vi "全局配置.vi"() -> ()   [LabVIEW 2018]
uses:
  Settings/Settings.ctl
  Acquisition/Hardware Configuration.ctl
  Acquisition/Signal Type.ctl
  Acquisition/Acquisition.lvlib
  Settings/Settings.lvlib
panel:
  in  "配置":T1 {"串口通信UI"."Format" items=["标准帧", "扩展帧"]; "串口通信UI"."Type" items=["数据帧", "远程帧"]; "串口通信UI"."ID" format="0x%x"; "串口通信UI"."Fliter" items=["接收所有类型"=1, "只接收标准帧"=2, "只接收扩展帧"=3]; "串口通信UI"."kBaudRate" items=["5k bps"=1, "10k bps"=2, "20k bps"=3, "40k bps"=4, "50k bps"=5, "80k bps"=6, "100k bps"=7, "125k bps"=8, "200k bps"=9, "250k bps"=10, "400k bps"=11, "500k bps"=12, "666k bps"=13, "800k bps"=14, "1000k bps"=15, "33.33k bps"=16, "66.66k bps"=17, "83.33k bps"=18]; "串口通信UI"."Mode" items=["正常工作", "仅侦听模式", "自测模式（环回）"]; "串口通信UI"."InitFlag" items=["使用界面设置参数"=1]; "串口通信UI"."AccMask" format="%08x"; "串口通信UI"."AccCode" format="%08x"; "串口通信UI"."Channel" items=["通道1", "通道2"]; "串口通信UI"."DevType" items=["USB-CAN"=3, "USB-CAN2"=4]; "安全报警UI"."操作 8" items=["产生报警信息（不发声），等待手动操作", "产生报警信息（发声），等待手动操作", "产生报警信息（不发声），自动刹车", "产生报警信息（发声），自动刹车", "产生报警信息（不发声），立即自动断电，开启泄放电阻", "产生报警信息（发声），立即自动断电，开启泄放电阻"]; "安全报警UI"."操作 7" items=["产生报警信息（不发声），等待手动操作", "产生报警信息（发声），等待手动操作", "产生报警信息（不发声），自动刹车", "产生报警信息（发声），自动刹车", "产生报警信息（不发声），立即自动断电，开启泄放电阻", "产生报警信息（发声），立即自动断电，开启泄放电阻"]; "安全报警UI"."操作 6" items=["产生报警信息（不发声），等待手动操作", "产生报警信息（发声），等待手动操作", "产生报警信息（不发声），自动刹车", "产生报警信息（发声），自动刹车", "产生报警信息（不发声），立即自动断电，开启泄放电阻", "产生报警信息（发声），立即自动断电，开启泄放电阻"]; "安全报警UI"."操作 5" items=["产生报警信息（不发声），等待手动操作", "产生报警信息（发声），等待手动操作", "产生报警信息（不发声），自动刹车", "产生报警信息（发声），自动刹车", "产生报警信息（不发声），立即自动断电，开启泄放电阻", "产生报警信息（发声），立即自动断电，开启泄放电阻"]; "安全报警UI"."操作 4" items=["产生报警信息（不发声），等待手动操作", "产生报警信息（发声），等待手动操作", "产生报警信息（不发声），自动刹车", "产生报警信息（发声），自动刹车", "产生报警信息（不发声），立即自动断电，开启泄放电阻", "产生报警信息（发声），立即自动断电，开启泄放电阻"]; "安全报警UI"."操作 3" items=["产生报警信息（不发声），等待手动操作", "产生报警信息（发声），等待手动操作", "产生报警信息（不发声），自动刹车", "产生报警信息（发声），自动刹车", "产生报警信息（不发声），立即自动断电，开启泄放电阻", "产生报警信息（发声），立即自动断电，开启泄放电阻"]; "安全报警UI"."操作 2" items=["产生报警信息（不发声），等待手动操作", "产生报警信息（发声），等待手动操作", "产生报警信息（不发声），自动刹车", "产生报警信息（发声），自动刹车", "产生报警信息（不发声），立即自动断电，开启泄放电阻", "产生报警信息（发声），立即自动断电，开启泄放电阻"]; "安全报警UI"."操作" items=["产生报警信息（不发声），等待手动操作", "产生报警信息（发声），等待手动操作", "产生报警信息（不发声），自动刹车", "产生报警信息（发声），自动刹车", "产生报警信息（不发声），立即自动断电，开启泄放电阻", "产生报警信息（发声），立即自动断电，开启泄放电阻"]}
  # "参数配置文件"
  # "输入数据文件"
  # "EHA电机"
  # "模拟电机"
  # "注：每次运行实验时销毁现有所有图像"
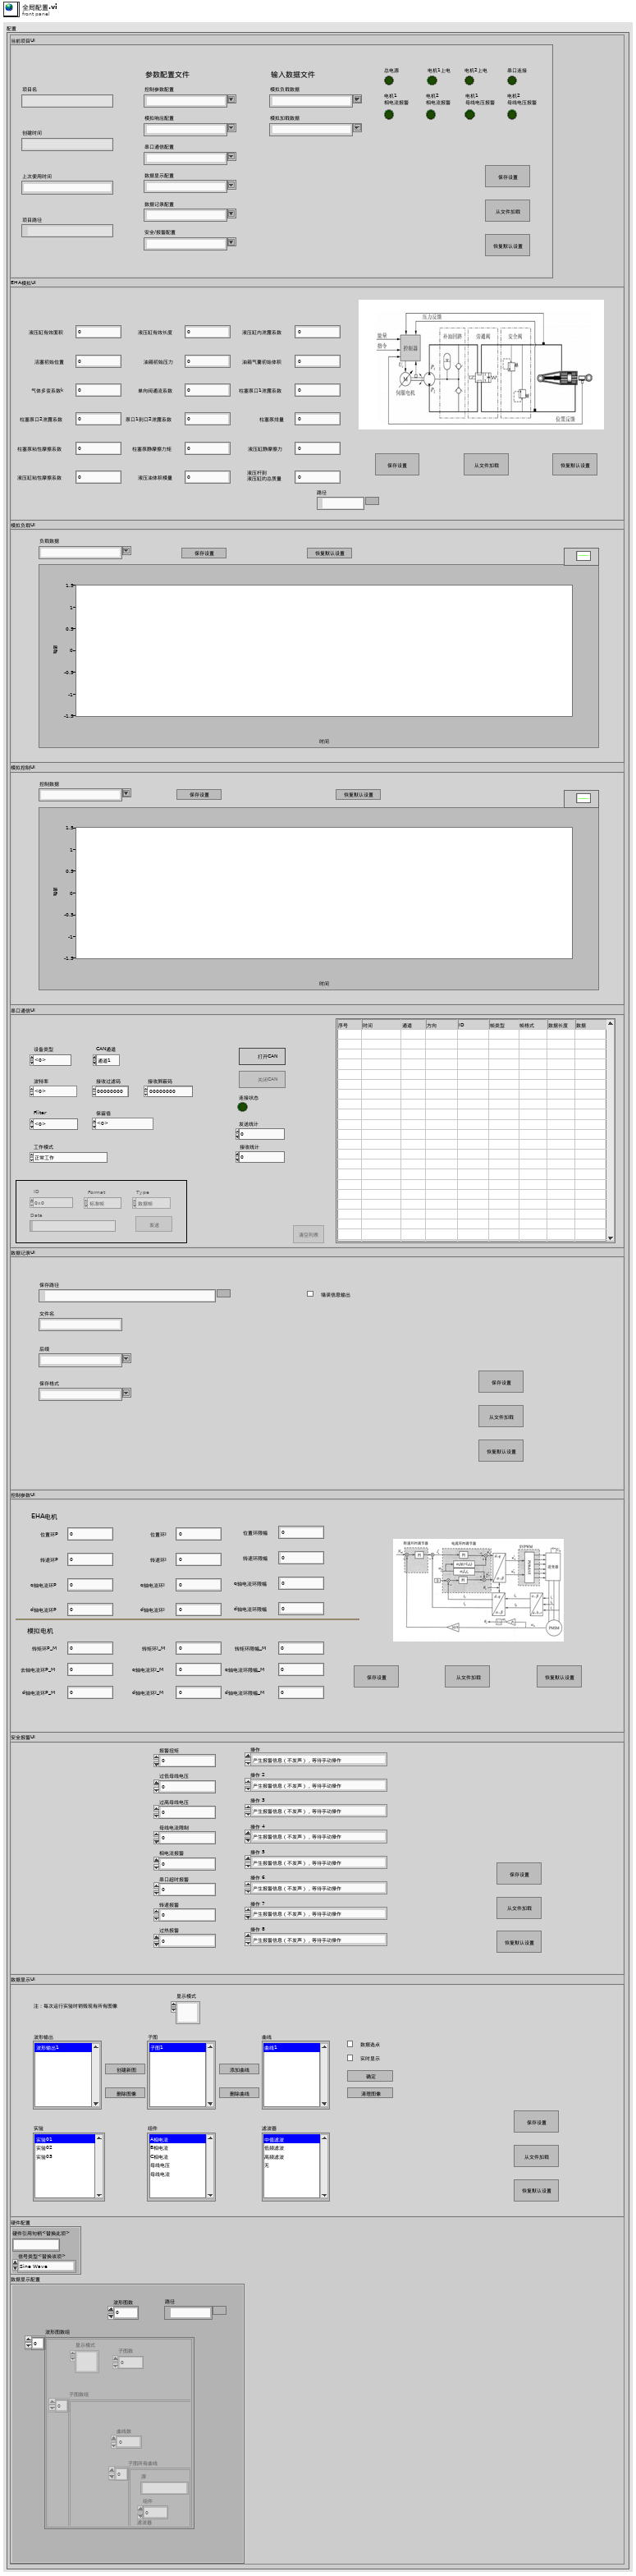
[diagram p1: front panel]
types:
  T1 = typedef "Settings.lvlib/Settings.ctl" = cluster{"当前项目UI":T2, "EHA模拟UI":T3, "模拟负载UI":T4, "模拟控制UI":T5, "串口通信UI":T6, "数据记录UI":T12, "控制参数UI":T13, "安全报警UI":T14, "数据显示UI":T15, "硬件配置":T16, "数据显示配置":T18}
  T2 = typedef "控件 5.ctl" = cluster{"控制参数配置":string, "模拟响应配置":string, "串口通信配置":string, "数据显示配置":string, "数据记录配置":string, "安全/报警配置":string, "模拟负载数据":string, "模拟加载数据":string, "总电源":bool, "电机1上电":bool, "电机2上电":bool, "串口连接":bool, "电机1\n相电流报警":bool, "电机2\n相电流报警":bool, "电机1\n母线电压报警":bool, "电机2\n母线电压报警":bool, "保存设置":bool, "从文件加载":bool, "恢复默认设置":bool, "路径":path, "项目路径":path, "项目名":string, "创建时间":string, "上次使用时间":string}
  T3 = typedef "EHA模拟UI.ctl" = cluster{"液压缸有效面积":dbl, "活塞初始位置":dbl, "气体多变系数k":dbl, "柱塞泵口2泄露系数":dbl, "柱塞泵粘性摩擦系数":dbl, "液压缸粘性摩擦系数":dbl, "液压缸有效长度":dbl, "油箱初始压力":dbl, "单向阀通流系数":dbl, "泵口1到口2泄露系数":dbl, "柱塞泵静摩擦力矩":dbl, "液压油体积模量":dbl, "保存设置":bool, "从文件加载":bool, "恢复默认设置":bool, "路径":path, "液压缸内泄露系数":dbl, "油箱气囊初始体积":dbl, "柱塞泵口1泄露系数":dbl, "柱塞泵排量":dbl, "液压缸静摩擦力":dbl, "液压杆到\n液压缸的总质量":dbl}
  T4 = typedef "控件 9.ctl" = cluster{"负载数据":string, "负载数据 2":waveform(dbl)[], "保存设置":bool, "恢复默认设置":bool}
  T5 = typedef "控件 7.ctl" = cluster{"控制数据":string, "负载数据 2":waveform(dbl)[], "保存设置":bool, "恢复默认设置":bool}
  T6 = typedef "控件 6.ctl" = cluster{"DevType":T7, "Channel":T8, "AccCode":u32, "AccMask":u32, "InitFlag":T9, "Mode":T10, "kBaudRate":u8, "Fliter":T11, "Open":bool, "Close":bool, "连接状态":bool, "SendCnt":u32, "RecvCnt":u32, "Send":bool, "ID":u32, "Data":string, "Type":u8, "Format":u8, "Clear":bool, "list":i32, "路径":path}
  T7 = typedef "ControlCAN.lvlib/DevType.ctl" = u32
  T8 = typedef "ControlCAN.lvlib/CAN Channel.ctl" = u32
  T9 = typedef "ControlCAN.lvlib/InitFlag.ctl" = u32
  T10 = typedef "ControlCAN.lvlib/Mode.ctl" = u8
  T11 = typedef "ControlCAN.lvlib/Fliter.ctl" = u8
  T12 = typedef "控件 3.ctl" = cluster{"保存路径":path, "文件名":string, "后缀":string, "保存格式":string, "复选框":bool, "保存设置":bool, "从文件加载":bool, "恢复默认设置":bool, "路径":path, "TDMS文件引用":refnum<k34>}
  T13 = typedef "控件 1.ctl" = cluster{"d轴电流环P_M":dbl, "转速环P":dbl, "q轴电流环P":dbl, "d轴电流环P":dbl, "转矩环P_M":dbl, "去轴电流环P_M":dbl, "转速环I":dbl, "q轴电流环I":dbl, "d轴电流环I":dbl, "转矩环I_M":dbl, "q轴电流环I_M":dbl, "d轴电流环I_M":dbl, "保存设置":bool, "从文件加载":bool, "恢复默认设置":bool, "路径":path, "位置环P":dbl, "位置环I":dbl, "转速环限幅":dbl, "q轴电流环限幅":dbl, "d轴电流环限幅":dbl, "位置环限幅":dbl, "转矩环限幅_M":dbl, "q轴电流环限幅_M":dbl, "d轴电流环限幅_M":dbl}
  T14 = typedef "控件 4.ctl" = cluster{"报警扭矩":dbl, "过低母线电压":dbl, "过高母线电压":dbl, "母线电流限制":dbl, "相电流报警":dbl, "串口超时报警":dbl, "转速报警":dbl, "过热报警":dbl, "操作":u16, "操作 2":u16, "操作 3":u16, "操作 4":u16, "操作 5":u16, "操作 6":u16, "操作 7":u16, "操作 8":u16, "保存设置":bool, "从文件加载":bool, "恢复默认设置":bool, "路径":path}
  T15 = typedef "控件 2.ctl" = cluster{"保存设置":bool, "从文件加载":bool, "恢复默认设置":bool, "实验":i32, "波形输出":i32, "组件":i32, "曲线":i32, "滤波器":i32, "删除曲线":bool, "清理图像":bool, "添加曲线":bool, "数据选点":bool, "确定按钮":bool, "实时显示":bool, "子图":i32, "显示模式":u16, "路径":path, "删除图像":bool, "创建新图":bool}
  T16 = typedef "Acquisition.lvlib/Hardware Configuration.ctl" = cluster{"硬件引用句柄<替换此项>":string, "信号类型<替换该项>":T17}
  T17 = typedef "Acquisition.lvlib/Signal Type.ctl" = enum16{"Sine Wave", "Square with Noise"}
  T18 = typedef "波形图簇.ctl" = cluster{"波形图数":u32, "波形图数组":T19[], "路径":path}
  T19 = typedef "波形图.ctl" = cluster{"显示模式":u16, "子图数":u32, "子图数组":T20[]}
  T20 = typedef "子图.ctl" = cluster{"子图所有曲线":T21[], "曲线数":u32}
  T21 = typedef "曲线簇.ctl" = cluster{"源":string, "组件":u32, "滤波器":u32}
diagram:
